vi "Command Line Target.vi"() -> ()   [LabVIEW 2023]
doc: "The VI is called from the command line based on a command line string generated by Passing Command Line Parameters.vi."
panel:
  out "Command Line Arguments":string[](array[string])
  out "String":string
  out "Numeric":dbl
  out "Boolean":bool
  # "When calling this VI from the command line, the Numeric, Boolean, and String values will be populated with command line parameter values. The Command Line Arguments array displays the arguments retrieved from the Application:Command Line Arguments property.\n\nNote: This VI must be set to Run when opened in order to retrieve the command line parameters properly. Go to File > VI Properties > Execution to set this property."
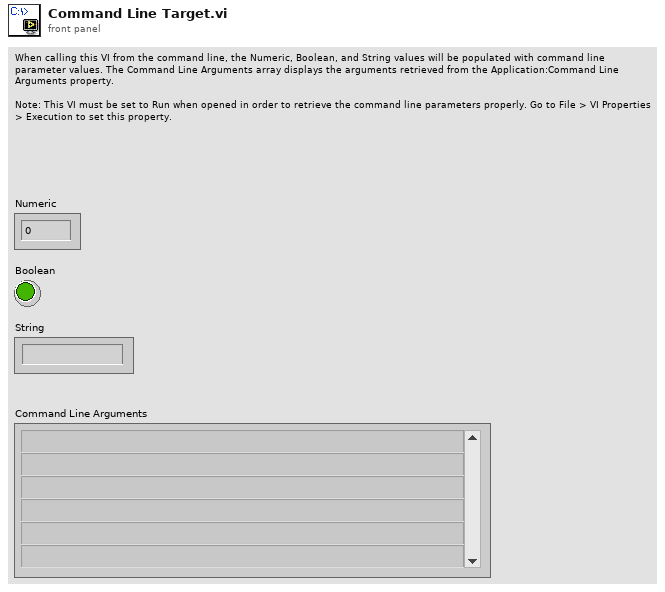
[diagram p1: front panel]
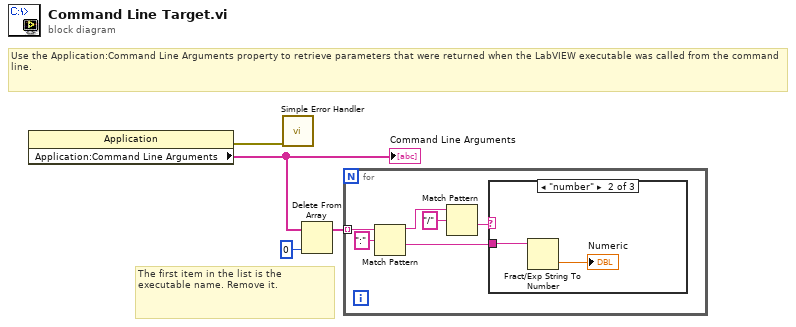
[diagram p0: block diagram]
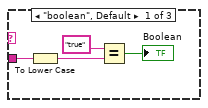
[diagram p2: hidden frame]
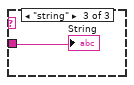
[diagram p3: hidden frame]
diagram:
  # "Use the Application:Command Line Arguments property to retrieve parameters that were returned when the LabVIEW executable was called from the command line."
  # "The first item in the list is the executable name. Remove it."
  n1 = property class="Application"() -> (error out=w1:errorcluster, "Application:Command Line Arguments"=w4:string[])  [unwired: 2 in, 1 out]
  "Command Line Arguments" <- w4
  n2 = call <vilib>:"Simple Error Handler.vi"("error in (no error)"=w1) -> ()  [unwired: 1 in, 8 out]
  n3 = Delete From Array(array=w4, index=0 ("length")) -> (array with subset deleted=w3:string[])  [unwired: 1 in, 1 out]
  n4 = for {
    tunnel: w3 -> [w9] mode=indexing
    n5 = Match Pattern(string=w9, regular expression=":") -> (before substring=w7:string, after substring=w8:string)  [unwired: 3 out]
    n6 = Match Pattern(string=w7, regular expression="/") -> (after substring=w5:string)  [unwired: 4 out]
    n7 = case shown="\"number\"" w5 {
      tunnel: w8 -> [w13 w16 w17]
      frame "boolean", Default {
        n8 = To Lower Case(string=w13) -> (all lower case string=w11:string)
        n9 = Equal?(x="true", y=w11) -> (x = y?=→"Boolean":bool)
      }
      frame "number" {
        n10 = Fract/Exp String To Number(string=w16) -> (number=→"Numeric":dbl)  [unwired: 4 out]
      }
      frame "string" {
        "String" <- w17
      }
    }
  }
